vi "周期启动 (子VI).vi"   [LabVIEW 2016, in "质控单元.lvlib"]
types:
  T1 = cluster{"是否启用仪器":bool, "CODMn":cluster{"启动测量模式":cluster{"测量模式":enum16{"水样测量", "标样核查", "加标回收", "平行样", "校零", "校标"}}, "确定按钮":bool}, "启动模块":cluster{"氨氮":bool, "总磷":bool, "总氮":bool, "CODMn":bool, "CODCr":bool}, "常规启动":bool, "直接启动":bool}
  T2 = cluster{"周期设置类型":enum16{"定点启动", "间隔启动"}, "定时功能启用":bool, "定时间隔":dbl, "间隔启动次数 ":dbl, "已经启动次数 ":dbl, "24H周期设置":bool[], "模块选择":cluster{"氨氮":bool, "总磷":bool, "总氮":bool, "CODMn":bool, "CODCr":bool}, "采配水启用":bool}
  T3 = typedef "LVDateTimeRec.ctl" = cluster{"秒数的小数部分":dbl, "秒":i32, "分":i32, "时":i32, "日":i32, "月":i32, "年":i32, "天数（周）":i32, "天数（年）":i32, "DST":i32}
  T4 = cluster{"氨氮":bool, "总磷":bool, "总氮":bool, "CODMn":bool, "CODCr":bool}
  T5 = enum32{"Bad", "Idle", "Run top level", "Running"}
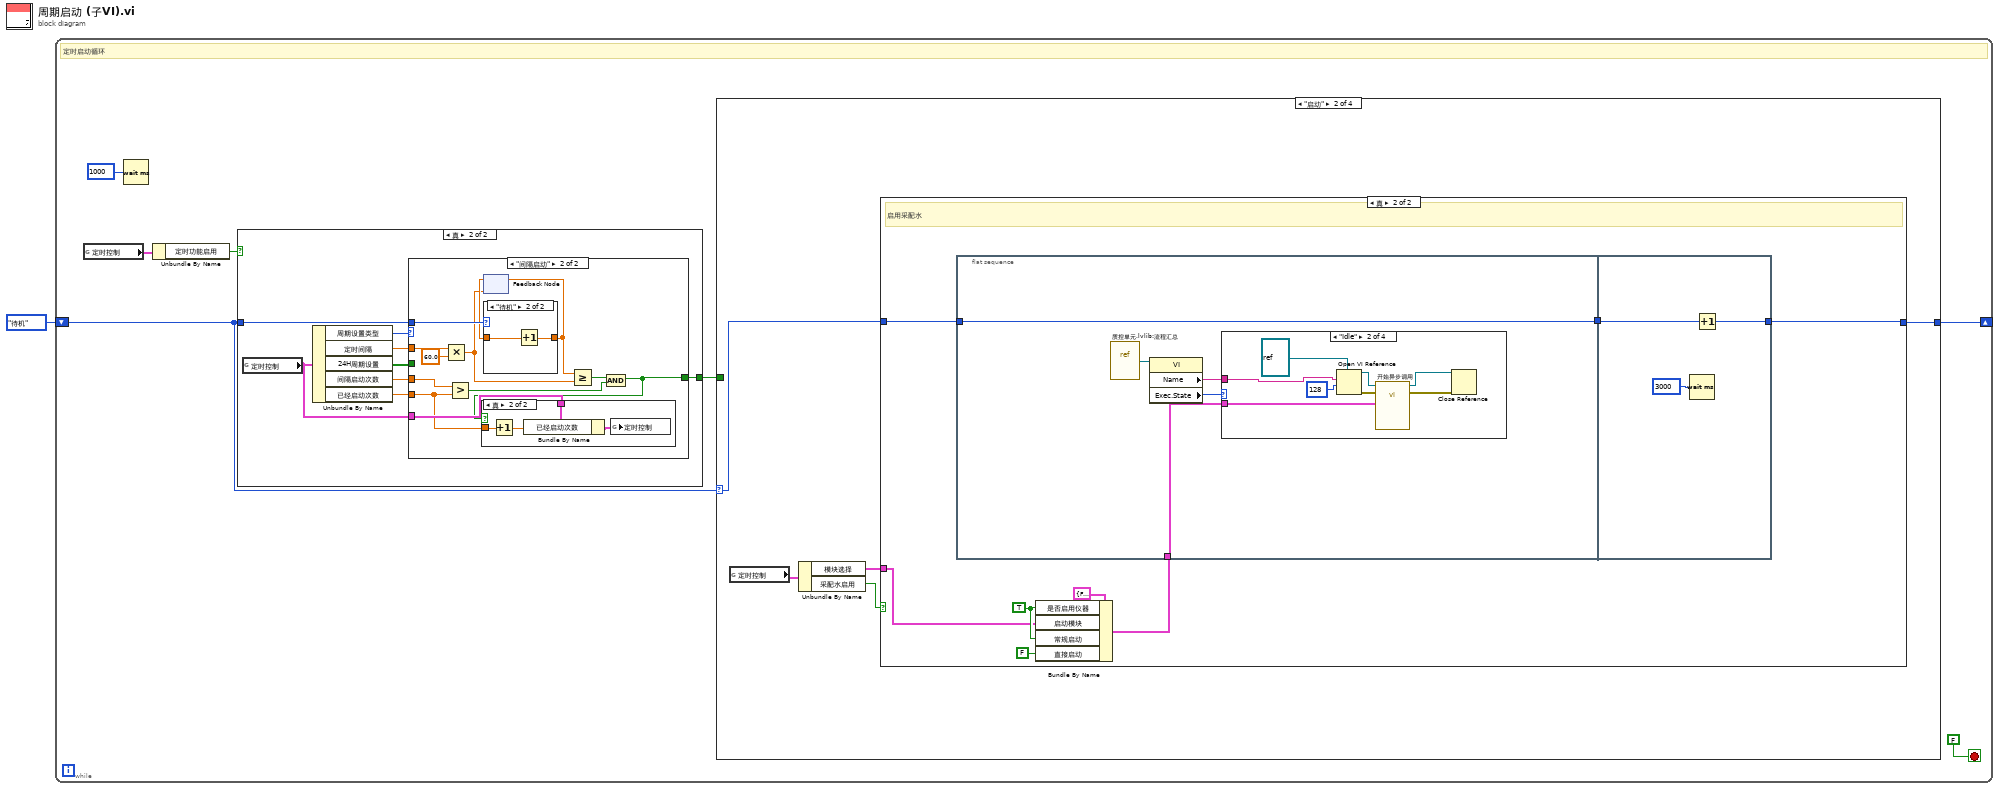
[diagram p0: block diagram]
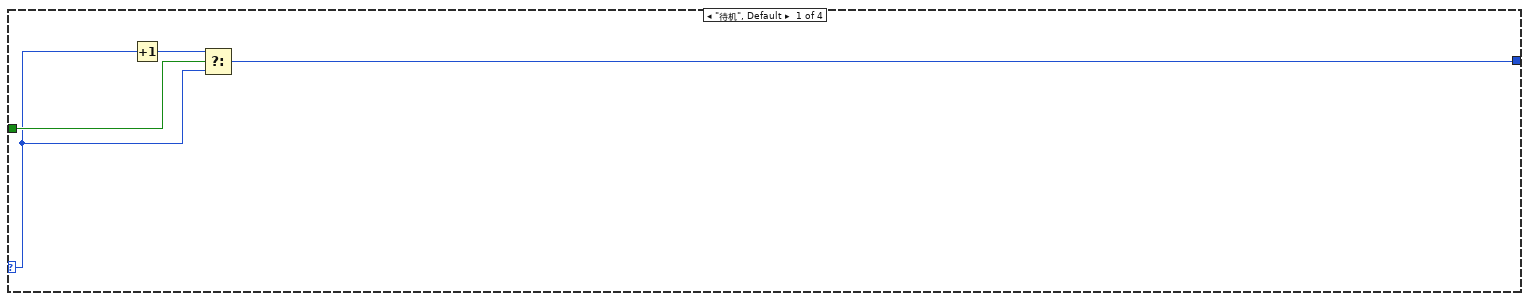
[diagram p2: hidden frame]
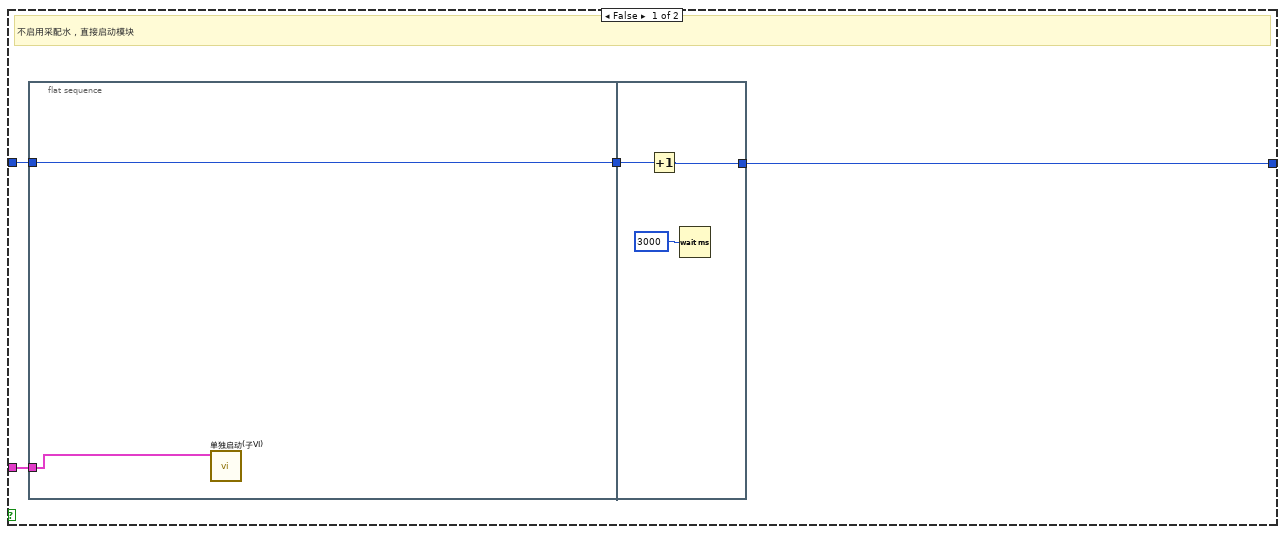
[diagram p3: hidden frame]
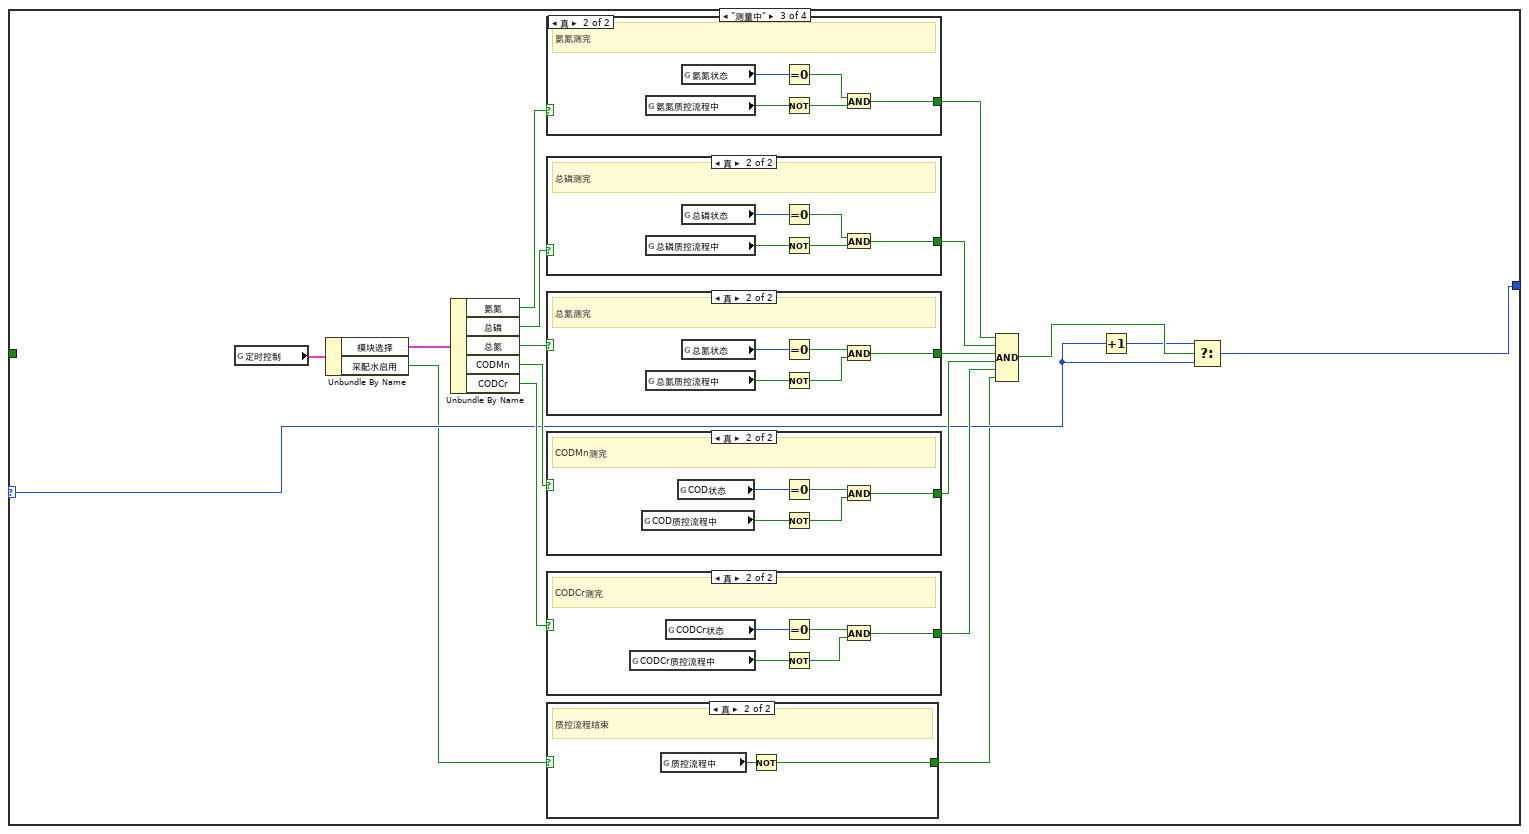
[diagram p7: hidden frame]
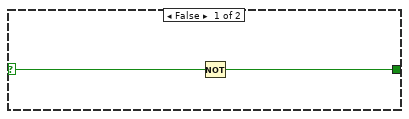
[diagram p8: hidden frame]
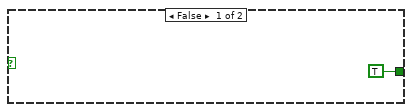
[diagram p9: hidden frame]
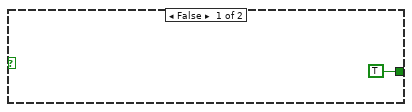
[diagram p10: hidden frame]
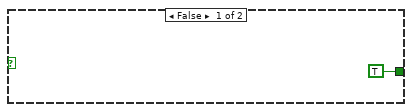
[diagram p11: hidden frame]
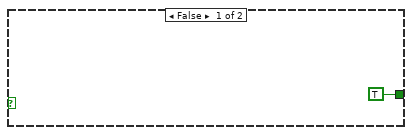
[diagram p12: hidden frame]
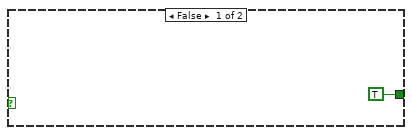
[diagram p13: hidden frame]
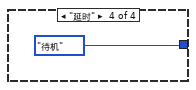
[diagram p14: hidden frame]
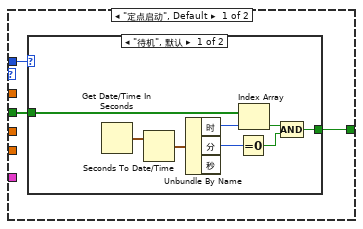
[diagram p16: hidden frame]
diagram:
  n1 = while {
    shift-right: [w6] -> _
    shift-left: enum16{"待机", "启动", "测量中", "延时"}."待机" -> [w5]
    stop <- FALSE stop-if-true
    # "定时启动循环"
    n2 = global read "断电保存全局.vi" "定时控制"() -> (w3:T2)
    n3 = Wait (ms)(milliseconds to wait=u32 1000 ("等待时间（毫秒）")) -> ()  [unwired: 1 out]
    n4 = Unbundle By Name(w3) -> ("定时功能启用"=w2:bool)
    n5 = case shown="真" w2 {
      tunnel: w5 -> [_ w108]
      tunnel: [_ w107] -> w4
      frame False {
      }
      frame True {
        n6 = global read "断电保存全局.vi" "定时控制"() -> (w104:T2)
        n7 = Unbundle By Name(w104) -> ("周期设置类型"=w109:enum16{"定点启动", "间隔启动"}, "定时间隔"=w110:dbl, "24H周期设置"=w111:bool[], "间隔启动次数"=w106:dbl, "已经启动次数"=w105:dbl)
        n8 = case shown="\"间隔启动\"" w109 {
          tunnel: w110 -> [_ w131]
          tunnel: w111 -> [w114 _]
          tunnel: w108 -> [w112 w134]
          tunnel: [w113 w123] -> w107
          tunnel: w106 -> [_ w127]
          tunnel: w105 -> [_ w124]
          tunnel: w104 -> [_ w125]
          frame "定点启动", Default {
            n9 = case shown="\"待机\", 默认" w112 {
              tunnel: w114 -> [w120 _]
              tunnel: [w115 _] -> w113
              frame "待机", Default {
                n10 = Get Date/Time In Seconds() -> (seconds since 1Jan1904=w122:timestamp)
                n11 = Seconds To Date/Time(time stamp (now)=w122) -> (date time rec=w121:T3)  [unwired: 1 in]
                n12 = Unbundle By Name(w121) -> ("时"=w119:i32, "分"=w118:i32)  [unwired: 1 out]
                n13 = Equal To 0?(x=w118) -> (x = 0?=w116:bool)
                n14 = Index Array(array=w120, index=w119) -> (element=w117:bool)
                n15 = Compound Arithmetic op=AND ("复合运算")(w117, w116) -> (w115:bool)
              }
              frame "启动" {
              }
            }
          }
          frame "间隔启动" {
            n16 = Multiply(x=w131, y=60.0) -> (x*y=w128:dbl)
            n17 = Greater?(x=w127, y=w124) -> (0:w126:bool)
            n18 = feedback #1(w128) -> (w133:dbl)
            n19 = case shown="\"待机\"" w134 {
              tunnel: w133 -> [_ w140]
              tunnel: [_ w139] -> w132
              frame Default {
              }
              frame "待机" {
                n20 = Increment(x=w140) -> (x+1=w139:dbl)
              }
            }
            n21 = feedback-in #1(w132) -> ()
            n22 = Greater Or Equal?(x=w132, y=w128) -> (x >= y?=w129:bool)
            n23 = And(x=w129, y=w126) -> (x .and. y?=w123:bool)
            n24 = case shown="真" w123 {
              tunnel: w125 -> [_ w138]
              tunnel: w124 -> [_ w137]
              frame False {
              }
              frame True {
                n25 = Increment(x=w137) -> (x+1=w136:dbl)
                n26 = Bundle By Name(cluster=w138, "已经启动次数"=w136) -> (w135:T2)
                n27 = global write "断电保存全局.vi" "定时控制"(w135) -> ()
              }
            }
          }
        }
      }
    }
    n28 = case shown="\"启动\"" w5 {
      selector: w5 -> [w9 w14 w54 _]
      tunnel: [w11 w17 w55 enum16{"待机", "启动", "测量中", "延时"}."待机"] -> w6
      tunnel: w4 -> [w12 _ _ _]
      frame "待机", Default {
        n29 = Increment(x=w9) -> (x+1=w10:enum16{"待机", "启动", "测量中", "延时"})
        n30 = Select(t=w10, s=w12, f=w9) -> (s? t:f=w11:enum16{"待机", "启动", "测量中", "延时"})
      }
      frame "启动" {
        n31 = global read "断电保存全局.vi" "定时控制"() -> (w15:T2)
        n32 = Unbundle By Name(w15) -> ("模块选择"=w16:T4, "采配水启用"=w13:bool)
        n33 = case shown="真" w13 {
          tunnel: [w20 w32] -> w17
          tunnel: w16 -> [w19 w28]
          tunnel: w14 -> [w18 w33]
          frame False {
            # "不启用采配水，直接启动模块"
            n34 = flat-sequence {
              tunnel: w19 -> [w22]
              tunnel: w18 -> [w23]
              tunnel: [w23] -> w21
              tunnel: [w26] -> w20
              tunnel: w21 -> [w25]
              frame #0 {
                n35 = call "单独启动(子VI).vi"("启动模块"=w22) -> ()  [unwired: 11 in]
              }
              frame #1 {
                n36 = Increment(x=w25) -> (x+1=w26:enum16{"待机", "启动", "测量中", "延时"})
                n37 = Wait (ms)(milliseconds to wait=u32 3000 ("等待时间（毫秒）")) -> ()  [unwired: 1 out]
              }
            }
          }
          frame True {
            w30 = TRUE ("是否启用仪器")
            # "启用采配水"
            n38 = flat-sequence {
              tunnel: [w39] -> w34
              tunnel: w33 -> [w39]
              tunnel: w27 -> [w35]
              tunnel: w34 -> [w50]
              tunnel: [w49] -> w32
              frame #0 {
                n39 = vi-ref "质控单元.lvlib:流程汇总.vi"() -> (w37:refnum<vi>)
                n40 = property class="VI"(reference=w37) -> ("Name"=w38:string, "Exec.State"=w36:T5)  [unwired: 1 in, 2 out]
                n41 = case shown="\"Idle\"" w36 {
                  tunnel: w38 -> [_ w46 _ _]
                  tunnel: w35 -> [_ w40 _ _]
                  frame "Bad", Default {
                  }
                  frame "Idle" {
                    n42 = Open VI Reference(type specifier VI Refnum (for type only)=refnum<vi> refnum ("类型说明符VI引用句柄（仅用于类型）"), vi path=w46, options=128 ("选项")) -> (vi reference=w47:refnum<vi>, error out=w43:errorcluster)  [unwired: 3 in]
                    n43 = call-by-ref "开始异步调用"(reference=w47, error in=w43, "参数"=w40) -> (reference out=w45:refnum<vi>, error out=w44:errorcluster)  [unwired: 11 in]
                    n44 = Close Reference(reference=w45, error in (no error)=w44) -> ()  [unwired: 1 out]
                  }
                  frame "Run top level" {
                  }
                  frame "Running" {
                  }
                }
              }
              frame #1 {
                n45 = Wait (ms)(milliseconds to wait=u32 3000 ("等待时间（毫秒）")) -> ()  [unwired: 1 out]
                n46 = Increment(x=w50) -> (x+1=w49:enum16{"待机", "启动", "测量中", "延时"})
              }
            }
            n47 = Bundle By Name(cluster=T1 {"是否启用仪器"=FALSE, "CODMn"={"启动测量模式"={"测量模式"=enum."水样测量"}, "确定按钮"=FALSE}, "启动模块"={"氨氮"=FALSE, "总磷"=FALSE, "总氮"=FALSE, "CODMn"=FALSE, "CODCr"=FALSE}, "常规启动"=FALSE, "直接启动"=FALSE} ("参数"), "是否启用仪器"=w30, "启动模块"=w28, "常规启动"=w30, "直接启动"=FALSE) -> (w27:T1)
          }
        }
      }
      frame "测量中" {
        n48 = global read "断电保存全局.vi" "定时控制"() -> (w68:T2)
        n49 = Unbundle By Name(w68) -> ("模块选择"=w67:T4, "采配水启用"=w53:bool)
        n50 = Unbundle By Name(w67) -> ("氨氮"=w60:bool, "总磷"=w59:bool, "总氮"=w58:bool, "CODMn"=w57:bool, "CODCr"=w56:bool)
        n51 = case shown="真" w60 {
          tunnel: [TRUE w100] -> w61
          frame False {
          }
          frame True {
            # "氨氮测完"
            n52 = global read "质控测完标志全局 1.vi" "氨氮质控流程中"() -> (w102:bool)
            n53 = global read "加标回收状态全局变量.vi" "氨氮状态"() -> (w99:u16)
            n54 = Equal To 0?(x=w99) -> (x = 0?=w98:bool)
            n55 = Not(x=w102) -> (.not. x?=w101:bool)
            n56 = And(x=w98, y=w101) -> (x .and. y?=w100:bool)
          }
        }
        n57 = case shown="真" w59 {
          tunnel: [TRUE w94] -> w62
          frame False {
          }
          frame True {
            # "总磷测完"
            n58 = global read "质控测完标志全局 1.vi" "总磷质控流程中"() -> (w96:bool)
            n59 = global read "加标回收状态全局变量.vi" "总磷状态"() -> (w93:u16)
            n60 = Equal To 0?(x=w93) -> (x = 0?=w92:bool)
            n61 = Not(x=w96) -> (.not. x?=w95:bool)
            n62 = And(x=w92, y=w95) -> (x .and. y?=w94:bool)
          }
        }
        n63 = case shown="真" w58 {
          tunnel: [TRUE w88] -> w63
          frame False {
          }
          frame True {
            # "总氮测完"
            n64 = global read "质控测完标志全局 1.vi" "总氮质控流程中"() -> (w90:bool)
            n65 = global read "加标回收状态全局变量.vi" "总氮状态"() -> (w87:u16)
            n66 = Equal To 0?(x=w87) -> (x = 0?=w86:bool)
            n67 = Not(x=w90) -> (.not. x?=w89:bool)
            n68 = And(x=w86, y=w89) -> (x .and. y?=w88:bool)
          }
        }
        n69 = case shown="真" w57 {
          tunnel: [TRUE w82] -> w64
          frame False {
          }
          frame True {
            # "CODMn测完"
            n70 = global read "质控测完标志全局 1.vi" "COD质控流程中"() -> (w84:bool)
            n71 = global read "加标回收状态全局变量.vi" "COD状态"() -> (w81:u16)
            n72 = Equal To 0?(x=w81) -> (x = 0?=w80:bool)
            n73 = Not(x=w84) -> (.not. x?=w83:bool)
            n74 = And(x=w80, y=w83) -> (x .and. y?=w82:bool)
          }
        }
        n75 = case shown="真" w56 {
          tunnel: [TRUE w76] -> w65
          frame False {
          }
          frame True {
            # "CODCr测完"
            n76 = global read "质控测完标志全局 1.vi" "CODCr质控流程中"() -> (w78:bool)
            n77 = global read "加标回收状态全局变量.vi" "CODCr状态"() -> (w75:u16)
            n78 = Equal To 0?(x=w75) -> (x = 0?=w74:bool)
            n79 = Not(x=w78) -> (.not. x?=w77:bool)
            n80 = And(x=w74, y=w77) -> (x .and. y?=w76:bool)
          }
        }
        n81 = case shown="真" w53 {
          selector: w53 -> [w70 _]
          tunnel: [w69 w71] -> w52
          frame False {
            n82 = Not(x=w70) -> (.not. x?=w69:bool)
          }
          frame True {
            # "质控流程结束"
            n83 = global read "质控测完标志全局 1.vi" "质控流程中"() -> (w72:bool)
            n84 = Not(x=w72) -> (.not. x?=w71:bool)
          }
        }
        n85 = Compound Arithmetic op=AND ("复合运算")(w61, w62, w63, w64, w65, w52) -> (w66:bool)
        n86 = Increment(x=w54) -> (x+1=w51:enum16{"待机", "启动", "测量中", "延时"})
        n87 = Select(t=w51, s=w66, f=w54) -> (s? t:f=w55:enum16{"待机", "启动", "测量中", "延时"})
      }
      frame "延时" {
      }
    }
  }
